vi "Autonomous Independent_old.vi"() -> ()   [LabVIEW 2011]
doc: "This VI is called when autonomous begins, and will automatically be terminated when autonomous ends. You can carry out timed or sensor driven robot movement independently without needing to return to the caller."
uses:
  <vilib>/Rock Robotics/WPI/Joystick/WPI_JoystickButtonState.ctl
  Robot Global Data.vi
  <vilib>/addons/control/pid/pid.llb/PID (DBL).vi
  <vilib>/Rock Robotics/WPI/RobotDrive/WPI_RobotDriveArcadeDrive_Standard(NoSaturation).vi
  <vilib>/addons/control/pid/NI_PID_pid.lvlib
panel:
  in  "ARM_FWD_LIMIT":dbl(slide)=0.4723926380368098 scale=1.0..-1.0
  in  "ARM_REV_LIMIT":dbl(slide)=-0.15950920245398775 scale=1.0..-1.0
  in  "ARM_HOME":dbl(slide)=0.47 scale=1.0..-1.0
  out "Kinect_Drive_Reduce":dbl=0.5
  out "KINECT_BTNS":T1
  out "LEFT_ARM_AXES":T2
  out "RIGHT_ARM_AXES":T2
  in  "Ball_Sucker_Speed":dbl=1.0
  in  "Feed_Speed_Cntrl":dbl=1.0
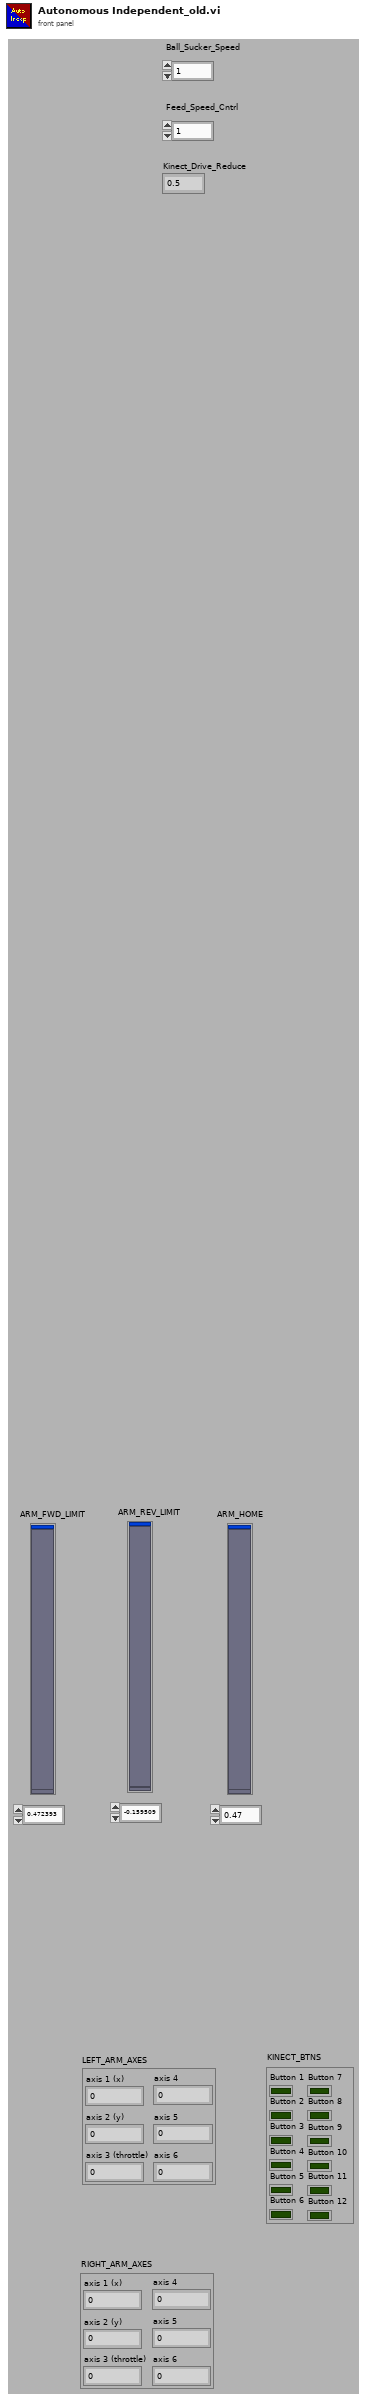
[diagram p1: front panel]
types:
  T1 = typedef "WPI_JoystickButtonState.ctl" = cluster{"Button 1":bool, "Button 2":bool, "Button 3":bool, "Button 4":bool, "Button 5":bool, "Button 6":bool, "Button 7":bool, "Button 8":bool, "Button 9":bool, "Button 10":bool, "Button 11":bool, "Button 12":bool}
  T2 = cluster{"axis 1 (x)":dbl, "axis 2 (y)":dbl, "axis 3 (throttle)":dbl, "axis 4":dbl, "axis 5":dbl, "axis 6":dbl}
  T3 = cluster{"proportional gain (Kc)":dbl, "integral time (Ti, min)":dbl, "derivative time (Td, min)":dbl}
  T4 = typedef "WPI_RobotDriveDevRef.ctl" = cluster{"DevStatus":errorcluster, "Motors[]":T5[], "Square Inputs":bool, "Max Output":dbl, "Isochronous":bool}
  T5 = typedef "WPI_MotorControlDeviceRef.ctl" = cluster{"DeviceStatus":errorcluster, "Type":enum16{"PWM", "CAN"}, "PWM":cluster{"Digital Module":T6, "PWM Channel":T7, "DeadBand":T8}, "CAN":cluster{"Device Number":u8, "Control Mode":T9, "Semaphore":T10, "Max Vout":dbl}, "Invert":bool, "TransformRef":T11, "InvTransformRef":T11}
  T6 = typedef "FPGA_TypedefDigitalModule.ctl" = enum16{"Digital Module 1", "Digital Module 2"}
  T7 = typedef "FPGA_DIOPWMChannel.ctl" = enum8{"PWM 1", "PWM 2", "PWM 3", "PWM 4", "PWM 5", "PWM 6", "PWM 7", "PWM 8", "PWM 9", "PWM 10", "Invalid"}
  T8 = typedef "WPI_PWMDeadband.ctl" = cluster{"Name":string, "maxPositivePwm":i32, "minPositivePwm":i32, "centerPwm":i32, "maxNegativePwm":i32, "minNegativePwm":i32, "angularRange":u16}
  T9 = typedef "WPI_CANJaguar_ControlMode.ctl" = enum8{"Percent VBus", "Current", "Speed", "Position", "Voltage"}
  T10 = typedef "Semaphore RefNum" = refnum<k1>
  T11 = typedef "WPI_PWMTransform_ConPane.ctl" = refnum<vi>
  T12 = typedef "WPI_JoystickDevRef.ctl" = cluster{"Device":T13}
  T13 = typedef "WPI_JoystickDeviceEnum.ctl" = enum16{"USB 1", "USB 2", "USB 3", "USB 4", "Kinect 1", "Kinect 2"}
  T14 = typedef "WPI_AnalogChannelDevRef.ctl" = cluster{"DevStatus":errorcluster, "Analog Module":T15, "Analog Channel":T16}
  T15 = typedef "FPGA_TypedefAnalogModule.ctl" = enum16{"Analog Module 1", "Analog Module 2"}
  T16 = typedef "FPGA_AIChannel.ctl" = enum8{"AI 1", "AI 2", "AI 3", "AI 4", "AI 5", "AI 6", "AI 7", "AI 8", "Invalid"}
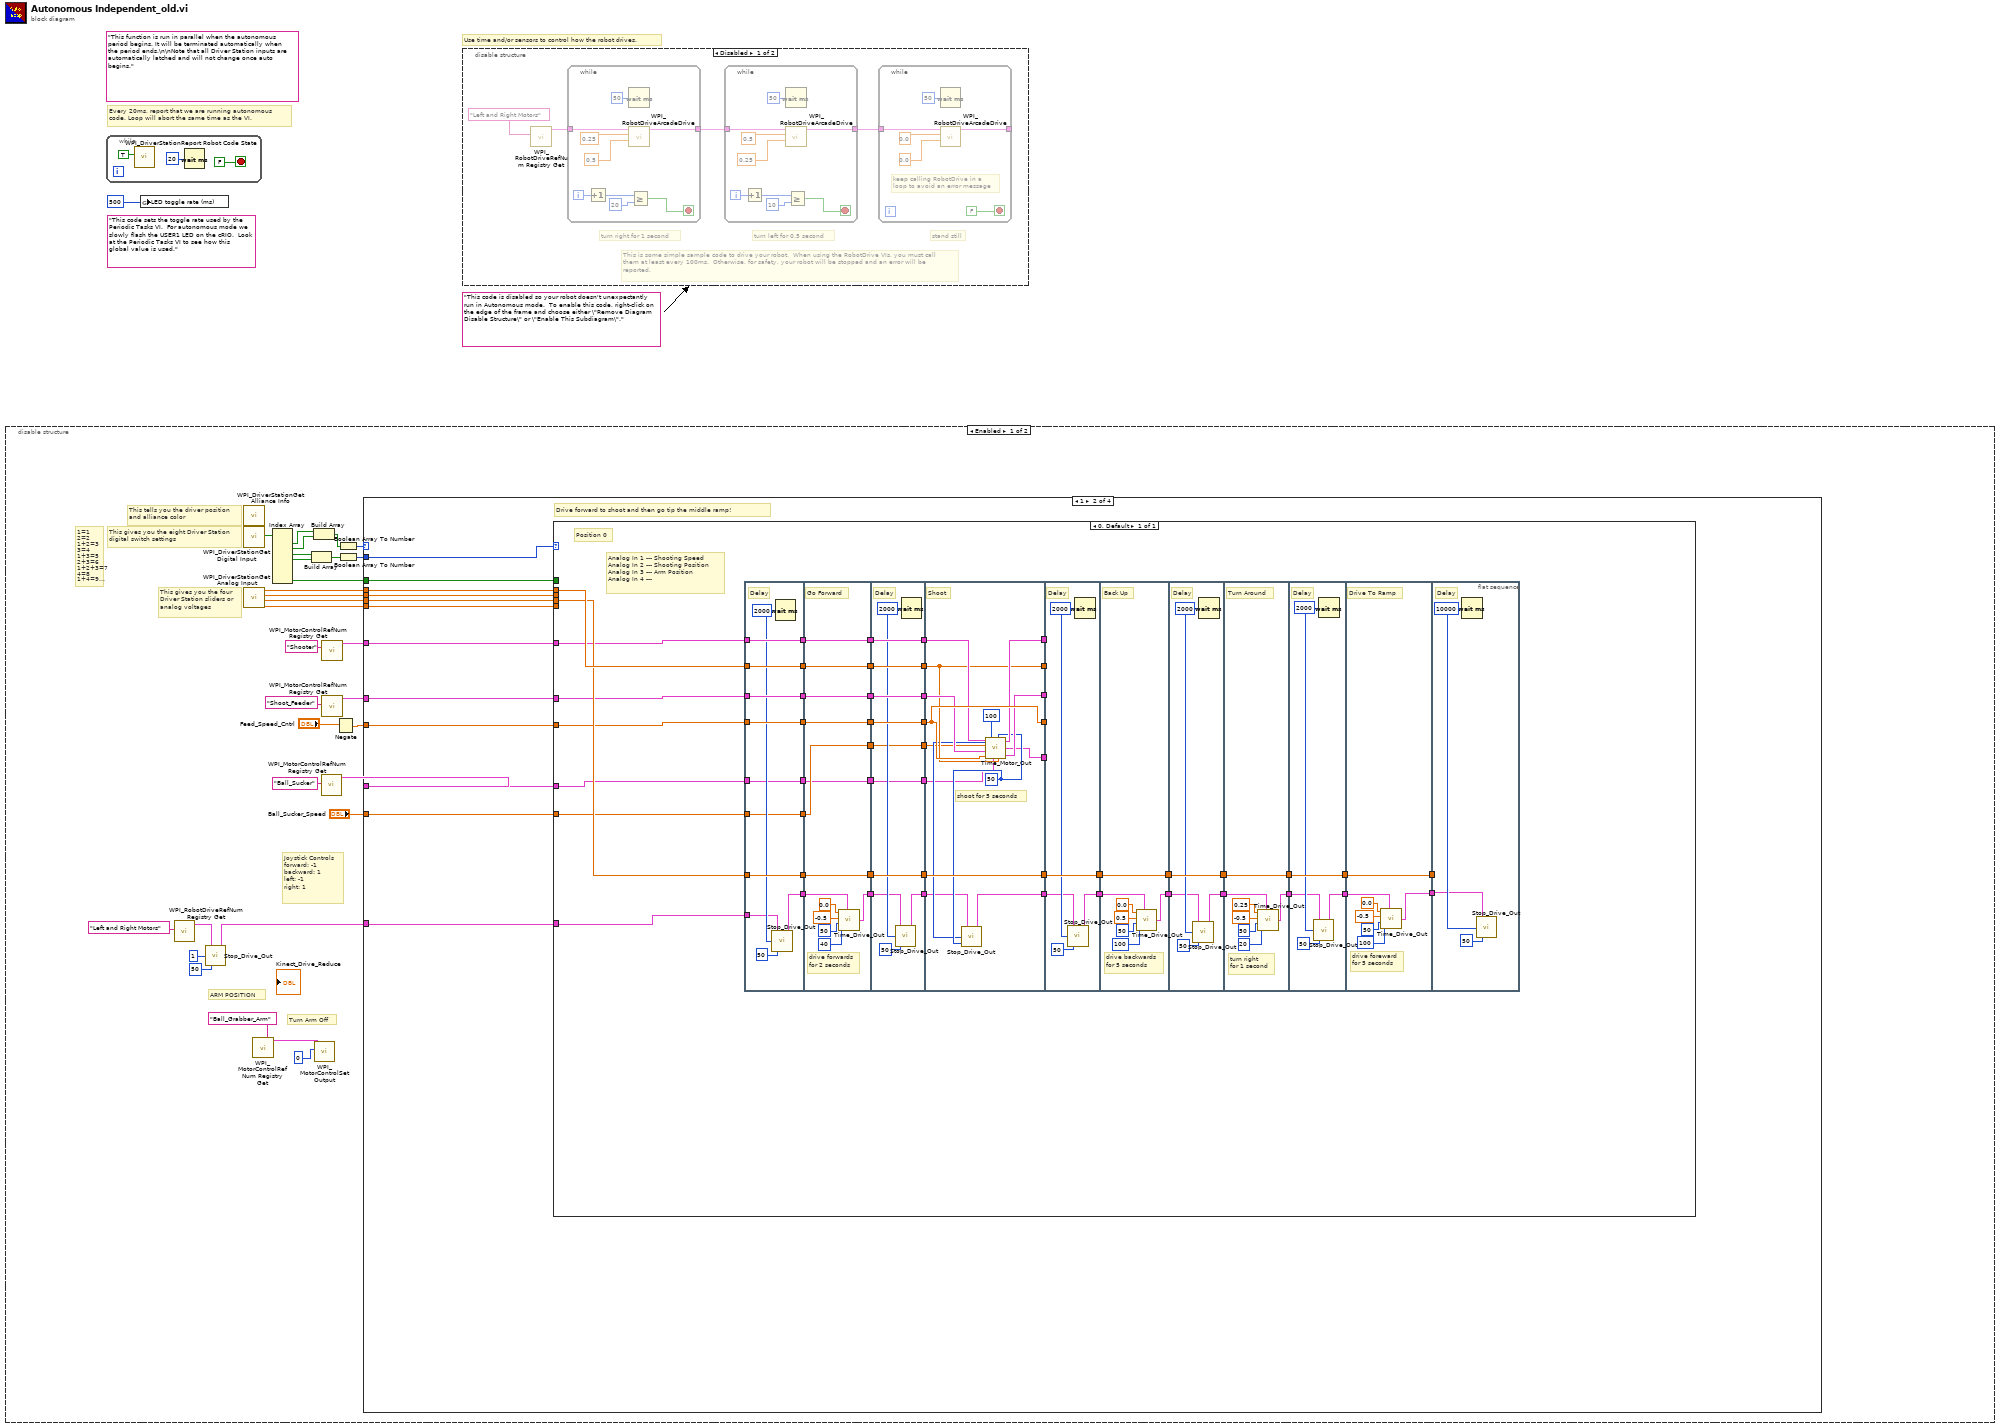
[diagram p0: block diagram]
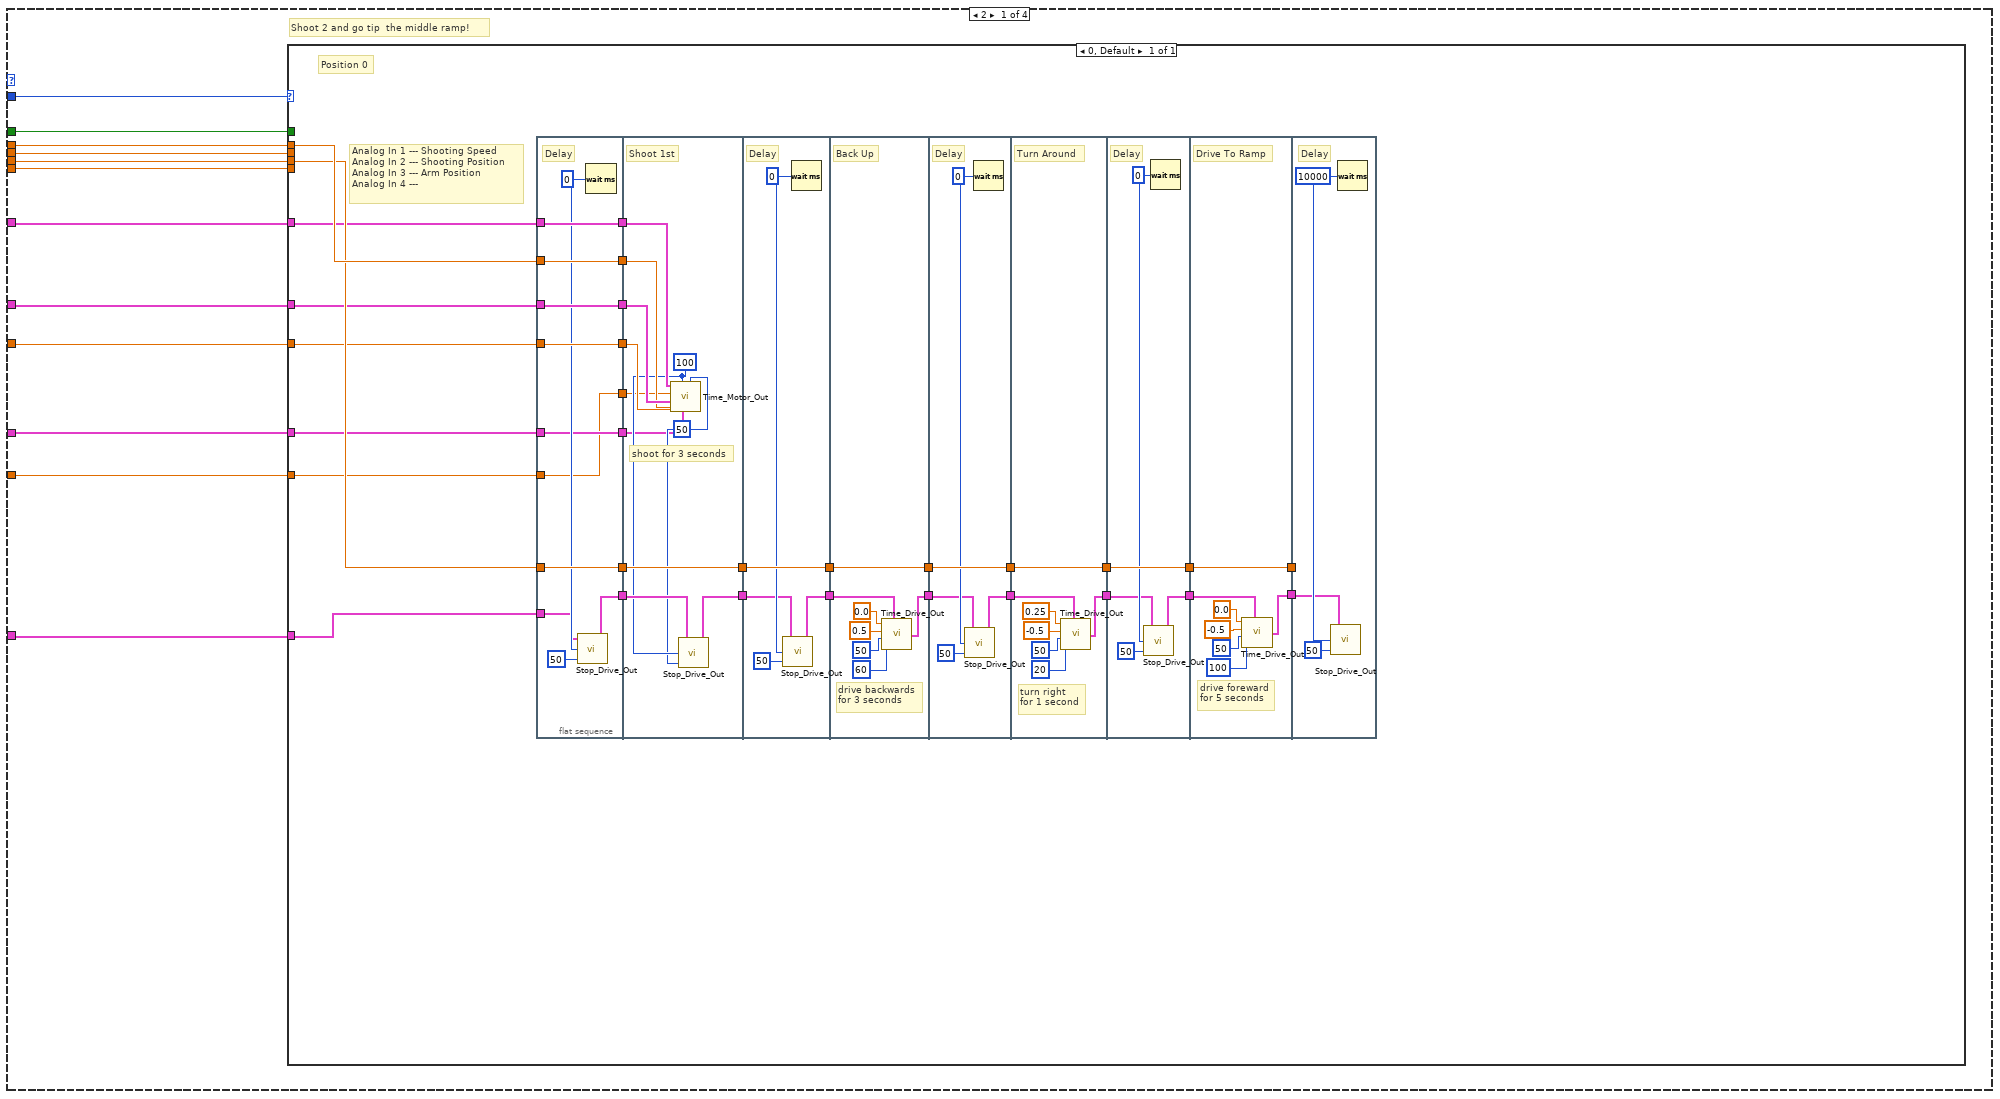
[diagram p2: hidden frame]
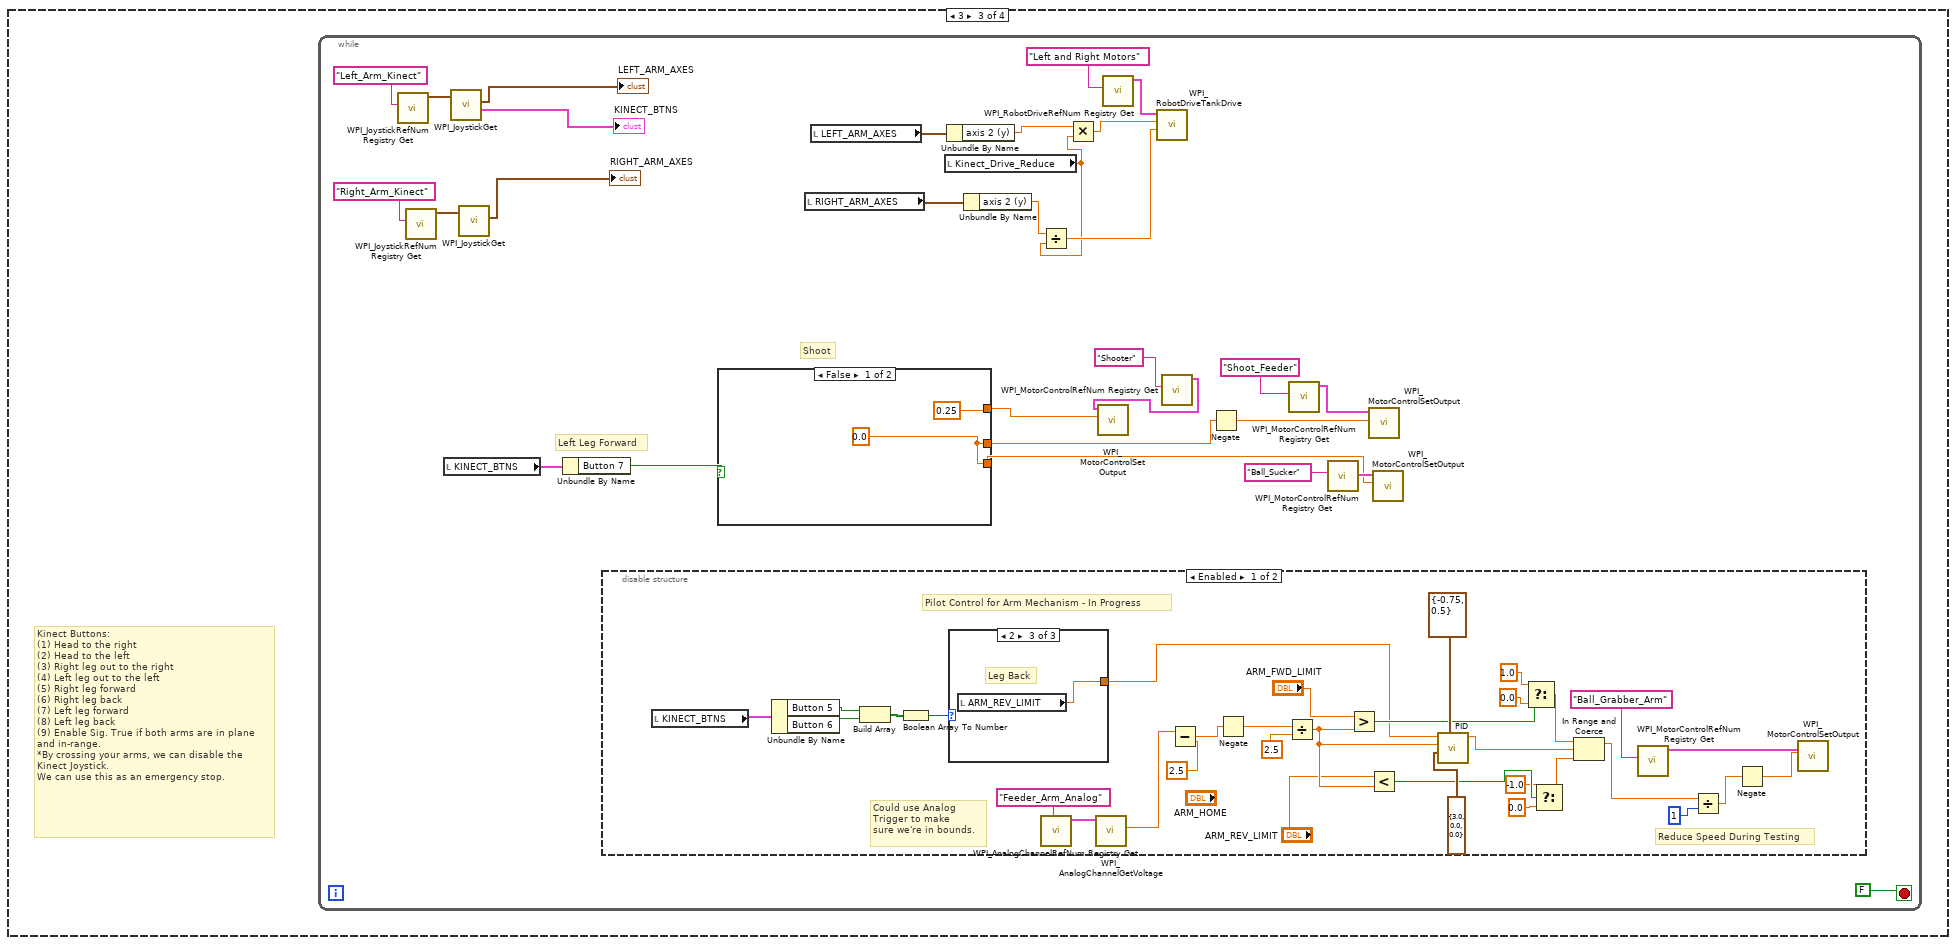
[diagram p3: hidden frame]
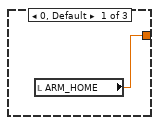
[diagram p4: hidden frame]
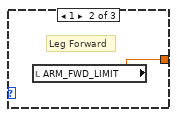
[diagram p5: hidden frame]
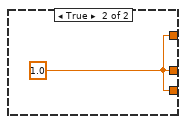
[diagram p7: hidden frame]
diagram:
  (unwired) "This code sets the toggle rate used by the Periodic Tasks VI.  For autonomous mode we slowly flash the USER1 LED on the cRIO.  Look at the Periodic Tasks VI to see how this global value is used."
  (unwired) "This code is disabled so your robot doesn't unexpectantly run in Autonomous mode.  To enable this code, right-click on the edge of the frame and choose either \"Remove Diagram Disable Structure\" or \"Enable This Subdiagram\"."
  (unwired) "This function is run in parallel when the autonomous period begins. It will be terminated automatically when the period ends.\n\nNote that all Driver Station inputs are automatically latched and will not change once auto begins."
  # "Every 20ms, report that we are running autonomous\ncode. Loop will abort the same time as the VI."
  # "Use time and/or sensors to control how the robot drives."
  n1 = disable-structure shown="Enabled" {
    frame Enabled {
      # "Turn Arm Off"
      # "ARM POSITION"
      # "Joystick Controls\nforward: -1\nbackward: 1\nleft: -1\nright: 1"
      # "1=1\n2=2\n1+2=3\n3=4\n1+3=5\n2+3=6\n1+2+3=7\n4=8\n1+4=9\n2+4=10\n1+2+4=11\n3+4=12\n1+3+4=13\n2+3+4=14\n1+2+3+4=15"
      # "This tells you the driver position\nand alliance color"
      # "This gives you the eight Driver Station\ndigital switch settings"
      # "This gives you the four\nDriver Station sliders or\nanalog voltages"
      n2 = call <vilib>:"WPI_RobotDriveRefNum Registry Get.vi"("refnum name"="Left and Right Motors") -> ("RobotDriveDevRef"=w13:T4)  [unwired: 1 in, 9 out]
      n3 = call "Stop_Drive_Out.vi"("Step_Duration_ms"=50, "Num_Steps"=u32 1 ("milliseconds to wait"), "Drive_In"=w13) -> ("Drive_Out"=w12:T4)
      n4 = call <vilib>:"WPI_DriverStationGet Alliance Info.vi"() -> ()  [unwired: 12 out]
      n5 = call <vilib>:"WPI_DriverStationGet Digital Input.vi"() -> ("Driver Station Digital Input (1-8)"=w32:bool[])  [unwired: 11 out]
      n6 = call <vilib>:"WPI_DriverStationGet Analog Input.vi"() -> ("Analog 4 (V)"=w29:dbl, "Analog 3 (V)"=w30:dbl, "Analog 2 (V)"=w16:dbl, "Analog 1 (V)"=w17:dbl)  [unwired: 8 out]
      n7 = call <vilib>:"WPI_MotorControlRefNum Registry Get.vi"("refnum name"="Ball_Grabber_Arm") -> ("MotorControlDevRef"=w4:T5)  [unwired: 1 in, 9 out]
      n8 = Index Array(array=w32) -> (element #1=w20:bool, element #2=w19:bool, element #3=w22:bool, element #4=w21:bool, element #8=w28:bool)  [unwired: 8 in, 3 out]
      n9 = Build Array(w22, w21) -> (w31:bool[])
      n10 = Build Array(w20, w19) -> (w18:bool[])
      n11 = call <vilib>:"WPI_MotorControlSetOutput.vi"("Output"=0, "MotorControlDevRef"=w4) -> ()  [unwired: 3 in, 7 out]
      n12 = call <vilib>:"WPI_MotorControlRefNum Registry Get.vi"("refnum name"="Ball_Sucker") -> ("MotorControlDevRef"=w6:T5)  [unwired: 9 in, 1 out]
      n13 = call <vilib>:"WPI_MotorControlRefNum Registry Get.vi"("refnum name"="Shooter") -> ("MotorControlDevRef"=w26:T5)  [unwired: 9 in, 1 out]
      n14 = call <vilib>:"WPI_MotorControlRefNum Registry Get.vi"("refnum name"="Shoot_Feeder") -> ("MotorControlDevRef"=w24:T5)  [unwired: 9 in, 1 out]
      n15 = Negate(x="Feed_Speed_Cntrl") -> (-x=w8:dbl)
      n16 = Boolean Array To Number(Boolean array=w18) -> (number=w11:u32)
      n17 = Boolean Array To Number(Boolean array=w31) -> (number=w10:u32)
      n18 = case shown="1" w11 {
        tunnel: w17 -> [w43 w146 _ _]
        tunnel: w16 -> [w42 w145 _ _]
        tunnel: w30 -> [w41 w144 _ _]
        tunnel: w29 -> [w40 w143 _ _]
        tunnel: w28 -> [w44 w147 _ _]
        tunnel: w8 -> [w39 w142 _ _]
        tunnel: w26 -> [w38 w141 _ _]
        tunnel: w24 -> [w37 w140 _ _]
        tunnel: w12 -> [w36 w139 _ _]
        tunnel: w10 -> [w35 w138 _ _]
        tunnel: w6 -> [w34 w137 _ _]
        tunnel: "Ball_Sucker_Speed" -> [w33 w136 _ _]
        frame 2 {
          # "Shoot 2 and go tip  the middle ramp!"
          n19 = case shown="0, Default" w35 {
            tunnel: w44 -> [_]
            tunnel: w43 -> [w74]
            tunnel: w42 -> [_]
            tunnel: w41 -> [w73]
            tunnel: w40 -> [_]
            tunnel: w39 -> [w72]
            tunnel: w38 -> [w71]
            tunnel: w37 -> [w70]
            tunnel: w36 -> [w69]
            tunnel: w34 -> [w45]
            tunnel: w33 -> [w68]
            frame 0, Default {
              # "Analog In 1 --- Shooting Speed\nAnalog In 2 --- Shooting Position\nAnalog In 3 --- Arm Position\nAnalog In 4 ---"
              # "Position 0"
              n20 = flat-sequence {
                tunnel: [w85] -> w67
                tunnel: [w84] -> w66
                tunnel: [w80] -> w65
                tunnel: [w83] -> w64
                tunnel: [w82] -> w63
                tunnel: [w81] -> w62
                tunnel: w71 -> [w85]
                tunnel: w70 -> [w84]
                tunnel: w74 -> [w83]
                tunnel: w72 -> [w82]
                tunnel: w73 -> [w81]
                tunnel: w69 -> [w77]
                tunnel: w45 -> [w76]
                tunnel: [w76] -> w61
                tunnel: [w75] -> w60
                tunnel: w68 -> [w75]
                tunnel: w67 -> [w96]
                tunnel: w66 -> [w95]
                tunnel: w65 -> [w91]
                tunnel: w64 -> [w93]
                tunnel: w63 -> [w94]
                tunnel: [w92] -> w59
                tunnel: w62 -> [w92]
                tunnel: [w88] -> w58
                tunnel: w61 -> [w87]
                tunnel: w60 -> [w86]
                tunnel: [w98] -> w57
                tunnel: [w101] -> w56
                tunnel: w59 -> [w101]
                tunnel: w58 -> [w97]
                tunnel: w57 -> [w104]
                tunnel: [w103] -> w55
                tunnel: w56 -> [w102]
                tunnel: [w102] -> w54
                tunnel: w55 -> [w110]
                tunnel: [w113] -> w53
                tunnel: w54 -> [w113]
                tunnel: [w109] -> w52
                tunnel: [w115] -> w51
                tunnel: [w114] -> w50
                tunnel: w53 -> [w114]
                tunnel: w52 -> [w116]
                tunnel: w51 -> [w122]
                tunnel: [w125] -> w49
                tunnel: w50 -> [w125]
                tunnel: [w121] -> w48
                tunnel: [w127] -> w47
                tunnel: [w126] -> w46
                tunnel: w49 -> [w126]
                tunnel: w48 -> [w128]
                tunnel: w47 -> [w133]
                tunnel: w46 -> [_]
                frame #0 {
                  w79 = u32 0 ("milliseconds to wait")
                  # "Delay"
                  n21 = call "Stop_Drive_Out.vi"("Step_Duration_ms"=u32 50 ("milliseconds to wait"), "Num_Steps"=w79, "Drive_In"=w77) -> ("Drive_Out"=w80:T4)
                  n22 = Wait (ms)(milliseconds to wait=w79) -> ()  [unwired: 1 out]
                }
                frame #1 {
                  w89 = 50
                  w90 = 100
                  # "shoot for 3 seconds"
                  # "Shoot 1st"
                  n23 = call "Time_Motor_Out.vi"("Motor_1_Speed"=w93, "Step_Duration_ms"=w89, "Motor_3"=w87, "Motor_2_Speed"=w94, "Motor_2"=w95, "Num_Steps"=w90, "Motor_3_Speed"=w86, "Motor_1"=w96) -> ()  [unwired: 3 out]
                  n24 = call "Stop_Drive_Out.vi"("Step_Duration_ms"=w89, "Num_Steps"=w90, "Drive_In"=w91) -> ("Drive_Out"=w88:T4)
                }
                frame #2 {
                  w99 = u32 0 ("milliseconds to wait")
                  # "Delay"
                  n25 = call "Stop_Drive_Out.vi"("Step_Duration_ms"=u32 50 ("milliseconds to wait"), "Num_Steps"=w99, "Drive_In"=w97) -> ("Drive_Out"=w98:T4)
                  n26 = Wait (ms)(milliseconds to wait=w99) -> ()  [unwired: 1 out]
                }
                frame #3 {
                  # "drive backwards\nfor 3 seconds"
                  # "Back Up"
                  n27 = call "Time_Drive_Out.vi"("X_Axis"=0.0 ("X axis value"), "Y_Axis"=0.5 ("X axis value"), "Step_Duration_ms"=u32 50 ("milliseconds to wait"), "Num_Steps"=60, "Drive_In"=w104) -> ("Drive_Out"=w103:T4)
                }
                frame #4 {
                  w111 = u32 0 ("milliseconds to wait")
                  # "Delay"
                  n28 = call "Stop_Drive_Out.vi"("Step_Duration_ms"=u32 50 ("milliseconds to wait"), "Num_Steps"=w111, "Drive_In"=w110) -> ("Drive_Out"=w109:T4)
                  n29 = Wait (ms)(milliseconds to wait=w111) -> ()  [unwired: 1 out]
                }
                frame #5 {
                  # "turn right\nfor 1 second"
                  # "Turn Around"
                  n30 = call "Time_Drive_Out.vi"("X_Axis"=0.25 ("X axis value"), "Y_Axis"=-0.5 ("X axis value"), "Step_Duration_ms"=u32 50 ("milliseconds to wait"), "Num_Steps"=20, "Drive_In"=w116) -> ("Drive_Out"=w115:T4)
                }
                frame #6 {
                  w123 = u32 0 ("milliseconds to wait")
                  # "Delay"
                  n31 = call "Stop_Drive_Out.vi"("Step_Duration_ms"=u32 50 ("milliseconds to wait"), "Num_Steps"=w123, "Drive_In"=w122) -> ("Drive_Out"=w121:T4)
                  n32 = Wait (ms)(milliseconds to wait=w123) -> ()  [unwired: 1 out]
                }
                frame #7 {
                  # "drive foreward\nfor 5 seconds"
                  # "Drive To Ramp"
                  n33 = call "Time_Drive_Out.vi"("X_Axis"=0.0 ("X axis value"), "Y_Axis"=-0.5 ("X axis value"), "Step_Duration_ms"=u32 50 ("milliseconds to wait"), "Num_Steps"=100, "Drive_In"=w128) -> ("Drive_Out"=w127:T4)
                }
                frame #8 {
                  w134 = u32 10000 ("milliseconds to wait")
                  # "Delay"
                  n34 = call "Stop_Drive_Out.vi"("Step_Duration_ms"=u32 50 ("milliseconds to wait"), "Num_Steps"=w134, "Drive_In"=w133) -> ()  [unwired: 1 out]
                  n35 = Wait (ms)(milliseconds to wait=w134) -> ()  [unwired: 1 out]
                }
              }
            }
          }
        }
        frame 1 {
          # "Drive forward to shoot and then go tip the middle ramp!"
          n36 = case shown="0, Default" w138 {
            tunnel: w147 -> [_]
            tunnel: w146 -> [w198]
            tunnel: w145 -> [_]
            tunnel: w144 -> [w197]
            tunnel: w143 -> [_]
            tunnel: w142 -> [w196]
            tunnel: w141 -> [w195]
            tunnel: w140 -> [w194]
            tunnel: w139 -> [w193]
            tunnel: w137 -> [w192]
            tunnel: w136 -> [w191]
            frame 0, Default {
              # "Analog In 1 --- Shooting Speed\nAnalog In 2 --- Shooting Position\nAnalog In 3 --- Arm Position\nAnalog In 4 ---"
              # "Position 0"
              n37 = flat-sequence {
                tunnel: [w202] -> w190
                tunnel: [w209] -> w189
                tunnel: [w208] -> w188
                tunnel: [w207] -> w187
                tunnel: [w206] -> w186
                tunnel: [w205] -> w185
                tunnel: w195 -> [w207]
                tunnel: w194 -> [w208]
                tunnel: w198 -> [w206]
                tunnel: w196 -> [w209]
                tunnel: w197 -> [w205]
                tunnel: w193 -> [w201]
                tunnel: [w200] -> w184
                tunnel: w191 -> [w200]
                tunnel: [w199] -> w183
                tunnel: w192 -> [w199]
                tunnel: w190 -> [w218]
                tunnel: [w217] -> w182
                tunnel: [w216] -> w181
                tunnel: w189 -> [w216]
                tunnel: [w215] -> w180
                tunnel: w188 -> [w215]
                tunnel: [w214] -> w179
                tunnel: w187 -> [w214]
                tunnel: [w213] -> w178
                tunnel: w186 -> [w213]
                tunnel: w185 -> [w212]
                tunnel: [w212] -> w177
                tunnel: w184 -> [w211]
                tunnel: [w211] -> w176
                tunnel: w183 -> [w210]
                tunnel: [w210] -> w175
                tunnel: w182 -> [w226]
                tunnel: [w225] -> w174
                tunnel: [w233] -> w173
                tunnel: [w232] -> w172
                tunnel: w181 -> [w232]
                tunnel: [w231] -> w171
                tunnel: w180 -> [w231]
                tunnel: [w230] -> w170
                tunnel: w179 -> [w230]
                tunnel: [w229] -> w169
                tunnel: w178 -> [w229]
                tunnel: w177 -> [w233]
                tunnel: [w224] -> w168
                tunnel: w176 -> [w224]
                tunnel: [w223] -> w167
                tunnel: w175 -> [w223]
                tunnel: w174 -> [w238]
                tunnel: [w237] -> w166
                tunnel: w173 -> [w247]
                tunnel: [w247] -> w165
                tunnel: w172 -> [w246]
                tunnel: [w246] -> w164
                tunnel: w171 -> [w245]
                tunnel: [w244] -> w163
                tunnel: [w243] -> w162
                tunnel: w170 -> [w242]
                tunnel: w169 -> [w241]
                tunnel: [w241] -> w161
                tunnel: [w236] -> w160
                tunnel: w168 -> [w235]
                tunnel: w167 -> [w234]
                tunnel: w166 -> [w249]
                tunnel: [w248] -> w159
                tunnel: w165 -> [w252]
                tunnel: [w252] -> w158
                tunnel: w164 -> [_]
                tunnel: w163 -> [_]
                tunnel: w162 -> [_]
                tunnel: w161 -> [_]
                tunnel: w160 -> [_]
                tunnel: w159 -> [w254]
                tunnel: [w253] -> w157
                tunnel: w158 -> [w259]
                tunnel: [w259] -> w156
                tunnel: w157 -> [w261]
                tunnel: w156 -> [w264]
                tunnel: [w264] -> w155
                tunnel: [w260] -> w154
                tunnel: [w266] -> w153
                tunnel: [w265] -> w152
                tunnel: w155 -> [w265]
                tunnel: w154 -> [w267]
                tunnel: w153 -> [w273]
                tunnel: [w272] -> w151
                tunnel: [w276] -> w150
                tunnel: w152 -> [w276]
                tunnel: w151 -> [w279]
                tunnel: [w278] -> w149
                tunnel: [w277] -> w148
                tunnel: w150 -> [w277]
                tunnel: w149 -> [w284]
                tunnel: w148 -> [_]
                frame #0 {
                  w203 = u32 2000 ("milliseconds to wait")
                  # "Delay"
                  n38 = call "Stop_Drive_Out.vi"("Step_Duration_ms"=50, "Num_Steps"=w203, "Drive_In"=w201) -> ("Drive_Out"=w202:T4)
                  n39 = Wait (ms)(milliseconds to wait=w203) -> ()  [unwired: 1 out]
                }
                frame #1 {
                  # "drive forwards\nfor 2 seconds"
                  # "Go Forward"
                  n40 = call "Time_Drive_Out.vi"("X_Axis"=0.0 ("X axis value"), "Y_Axis"=-0.5 ("X axis value"), "Step_Duration_ms"=u32 50 ("milliseconds to wait"), "Num_Steps"=40, "Drive_In"=w218) -> ("Drive_Out"=w217:T4)
                }
                frame #2 {
                  w227 = u32 2000 ("milliseconds to wait")
                  # "Delay"
                  n41 = call "Stop_Drive_Out.vi"("Step_Duration_ms"=50, "Num_Steps"=w227, "Drive_In"=w226) -> ("Drive_Out"=w225:T4)
                  n42 = Wait (ms)(milliseconds to wait=w227) -> ()  [unwired: 1 out]
                }
                frame #3 {
                  w240 = 50
                  w239 = 100
                  # "Shoot"
                  # "shoot for 5 seconds"
                  n43 = call "Stop_Drive_Out.vi"("Step_Duration_ms"=w240, "Num_Steps"=w239, "Drive_In"=w238) -> ("Drive_Out"=w237:T4)
                  n44 = call "Time_Motor_Out.vi"("Motor_1_Speed"=w241, "Step_Duration_ms"=w240, "Motor_3"=w234, "Motor_2_Speed"=w246, "Motor_2"=w245, "Num_Steps"=w239, "Motor_3_Speed"=w235, "Motor_1"=w242) -> ("Motor_2_Out"=w244:T5, "Motor_3_Out"=w236:T5, "Motor_1_Out"=w243:T5)
                }
                frame #4 {
                  w250 = u32 2000 ("milliseconds to wait")
                  # "Delay"
                  n45 = call "Stop_Drive_Out.vi"("Step_Duration_ms"=50, "Num_Steps"=w250, "Drive_In"=w249) -> ("Drive_Out"=w248:T4)
                  n46 = Wait (ms)(milliseconds to wait=w250) -> ()  [unwired: 1 out]
                }
                frame #5 {
                  # "Back Up"
                  # "drive backwards\nfor 5 seconds"
                  n47 = call "Time_Drive_Out.vi"("X_Axis"=0.0 ("X axis value"), "Y_Axis"=0.5 ("X axis value"), "Step_Duration_ms"=u32 50 ("milliseconds to wait"), "Num_Steps"=100, "Drive_In"=w254) -> ("Drive_Out"=w253:T4)
                }
                frame #6 {
                  w262 = u32 2000 ("milliseconds to wait")
                  # "Delay"
                  n48 = call "Stop_Drive_Out.vi"("Step_Duration_ms"=50, "Num_Steps"=w262, "Drive_In"=w261) -> ("Drive_Out"=w260:T4)
                  n49 = Wait (ms)(milliseconds to wait=w262) -> ()  [unwired: 1 out]
                }
                frame #7 {
                  # "turn right\nfor 1 second"
                  # "Turn Around"
                  n50 = call "Time_Drive_Out.vi"("X_Axis"=0.25 ("X axis value"), "Y_Axis"=-0.5 ("X axis value"), "Step_Duration_ms"=u32 50 ("milliseconds to wait"), "Num_Steps"=20, "Drive_In"=w267) -> ("Drive_Out"=w266:T4)
                }
                frame #8 {
                  w274 = u32 2000 ("milliseconds to wait")
                  # "Delay"
                  n51 = call "Stop_Drive_Out.vi"("Step_Duration_ms"=50, "Num_Steps"=w274, "Drive_In"=w273) -> ("Drive_Out"=w272:T4)
                  n52 = Wait (ms)(milliseconds to wait=w274) -> ()  [unwired: 1 out]
                }
                frame #9 {
                  # "drive foreward\nfor 5 seconds"
                  # "Drive To Ramp"
                  n53 = call "Time_Drive_Out.vi"("X_Axis"=0.0 ("X axis value"), "Y_Axis"=-0.5 ("X axis value"), "Step_Duration_ms"=u32 50 ("milliseconds to wait"), "Num_Steps"=100, "Drive_In"=w279) -> ("Drive_Out"=w278:T4)
                }
                frame #10 {
                  w285 = u32 10000 ("milliseconds to wait")
                  # "Delay"
                  n54 = Wait (ms)(milliseconds to wait=w285) -> ()  [unwired: 1 out]
                  n55 = call "Stop_Drive_Out.vi"("Step_Duration_ms"=50, "Num_Steps"=w285, "Drive_In"=w284) -> ()  [unwired: 1 out]
                }
              }
            }
          }
        }
        frame 3 {
          # "Kinect Buttons:\n(1) Head to the right\n(2) Head to the left\n(3) Right leg out to the right\n(4) Left leg out to the left\n(5) Right leg forward\n(6) Right leg back\n(7) Left leg forward\n(8) Left leg back\n(9) Enable Sig. True if both arms are in plane and in-range.\n*By crossing your arms, we can disable the Kinect Joystick. \nWe can use this as an emergency stop."
          n56 = while {
            stop <- FALSE stop-if-true
            # "Left Leg Forward"
            # "Shoot"
            n57 = call <vilib>:"WPI_JoystickRefNum Registry Get.vi"("refnum name"="Left_Arm_Kinect") -> ("JoystickDevRef"=w312:T12)  [unwired: 1 in, 9 out]
            n58 = call <vilib>:"WPI_JoystickRefNum Registry Get.vi"("refnum name"="Right_Arm_Kinect") -> ("JoystickDevRef"=w310:T12)  [unwired: 1 in, 9 out]
            n59 = local read "KINECT_BTNS"() -> (w299:T1)
            n60 = call <vilib>:"WPI_JoystickGet.vi"("JoystickDevRef"=w312) -> ("Buttons"=→"KINECT_BTNS":T1, "Axes"=→"LEFT_ARM_AXES":T2)  [unwired: 1 in, 4 out]
            n61 = call <vilib>:"WPI_JoystickGet.vi"("JoystickDevRef"=w310) -> ("Axes"=→"RIGHT_ARM_AXES":T2)  [unwired: 1 in, 5 out]
            n62 = Unbundle By Name(w299) -> ("Button 7"=w298:bool)
            n63 = disable-structure shown="Enabled" {
              frame Enabled {
                # "Could use Analog\nTrigger to make \nsure we're in bounds."
                # "Reduce Speed During Testing"
                # "Pilot Control for Arm Mechanism - In Progress"
                n64 = local read "KINECT_BTNS"() -> (w320:T1)
                n65 = Unbundle By Name(w320) -> ("Button 5"=w317:bool, "Button 6"=w316:bool)
                n66 = Build Array(w317, w316) -> (w318:bool[])
                n67 = Boolean Array To Number(Boolean array=w318) -> (number=w319:u32)
                n68 = case shown="2" w319 {
                  tunnel: [w349 w350 w351] -> w326
                  frame 0, Default {
                    n69 = local read "ARM_HOME"() -> (w349:dbl)
                  }
                  frame 1 {
                    # "Leg Forward"
                    n70 = local read "ARM_FWD_LIMIT"() -> (w350:dbl)
                  }
                  frame 2 {
                    # "Leg Back"
                    n71 = local read "ARM_REV_LIMIT"() -> (w351:dbl)
                  }
                }
                n72 = call <vilib>:"WPI_AnalogChannelRefNum Registry Get.vi"("refnum name"="Feeder_Arm_Analog") -> ("AIDeviceRef"=w347:T14)  [unwired: 1 in, 9 out]
                n73 = call <vilib>:"WPI_AnalogChannelGetVoltage.vi"("AIDeviceRef"=w347) -> ("Voltage"=w344:dbl)  [unwired: 1 in, 9 out]
                n74 = Subtract(x=w344, y=2.5) -> (x-y=w321:dbl)
                n75 = Negate(x=w321) -> (-x=w322:dbl)
                n76 = Divide(x=w322, y=2.5) -> (x/y=w332:dbl)
                n77 = Greater?(x="ARM_FWD_LIMIT", y=w332) -> (0:w339:bool)
                n78 = Less?(x="ARM_REV_LIMIT", y=w332) -> (x < y?=w341:bool)
                n79 = call-poly <vilib>:"PID.vi"("output range"=cluster{"output low":dbl, "output high":dbl} {"output low"=-0.75, "output high"=0.5}, "PID gains"=T3 {"proportional gain (Kc)"=3.0, "integral time (Ti, min)"=0.0, "derivative time (Td, min)"=0.0}, "process variable"=w332, "setpoint"=w326) -> ("output"=w331:dbl)  [unwired: 2 in, 5 out]
                n80 = Select(t=1.0, s=w339, f=0.0) -> (s? t:f=w337:dbl)
                n81 = Select(t=-1.0, s=w341, f=0.0) -> (s? t:f=w338:dbl)
                n82 = In Range and Coerce(upper limit=w337, x=w331, lower limit=w338) -> (coerced(x)=w328:dbl)  [unwired: 1 out]
                n83 = call <vilib>:"WPI_MotorControlRefNum Registry Get.vi"("refnum name"="Ball_Grabber_Arm") -> ("MotorControlDevRef"=w348:T5)  [unwired: 1 in, 9 out]
                n84 = Divide(x=w328, y=1) -> (x/y=w324:dbl)
                n85 = Negate(x=w324) -> (-x=w323:dbl)
                n86 = call <vilib>:"WPI_MotorControlSetOutput.vi"("Output"=w323, "MotorControlDevRef"=w348) -> ()  [unwired: 3 in, 7 out]
              }
              frame Disabled {
              }
            }
            n87 = case shown="False" w298 {
              tunnel: [0.25 w354] -> w290
              tunnel: [w353 w354] -> w289
              tunnel: [w353 w354] -> w288
              frame False {
                w353 = 0.0
              }
              frame True {
                w354 = 1.0
              }
            }
            n88 = local read "RIGHT_ARM_AXES"() -> (w303:T2)
            n89 = local read "LEFT_ARM_AXES"() -> (w306:T2)
            n90 = local read "Kinect_Drive_Reduce"() -> (w300:dbl)
            n91 = Unbundle By Name(w306) -> ("axis 2 (y)"=w305:dbl)
            n92 = Unbundle By Name(w303) -> ("axis 2 (y)"=w302:dbl)
            n93 = Divide(x=w302, y=w300) -> (x/y=w301:dbl)
            n94 = Multiply(x=w305, y=w300) -> (x*y=w304:dbl)
            n95 = call <vilib>:"WPI_RobotDriveRefNum Registry Get.vi"("refnum name"="Left and Right Motors") -> ("RobotDriveDevRef"=w307:T4)  [unwired: 1 in, 9 out]
            n96 = call <vilib>:"WPI_RobotDriveTankDrive.vi"("Right axis value"=w301, "Left axis value"=w304, "RobotDriveDevRef"=w307) -> ()  [unwired: 7 in, 2 out]
            n97 = call <vilib>:"WPI_MotorControlRefNum Registry Get.vi"("refnum name"="Shooter") -> ("MotorControlDevRef"=w296:T5)  [unwired: 9 in, 1 out]
            n98 = call <vilib>:"WPI_MotorControlSetOutput.vi"("Output"=w290, "MotorControlDevRef"=w296) -> ()  [unwired: 8 in, 2 out]
            n99 = Negate(x=w289) -> (-x=w293:dbl)
            n100 = call <vilib>:"WPI_MotorControlRefNum Registry Get.vi"("refnum name"="Shoot_Feeder") -> ("MotorControlDevRef"=w294:T5)  [unwired: 9 in, 1 out]
            n101 = call <vilib>:"WPI_MotorControlRefNum Registry Get.vi"("refnum name"="Ball_Sucker") -> ("MotorControlDevRef"=w291:T5)  [unwired: 9 in, 1 out]
            n102 = call <vilib>:"WPI_MotorControlSetOutput.vi"("Output"=w293, "MotorControlDevRef"=w294) -> ()  [unwired: 8 in, 2 out]
            n103 = call <vilib>:"WPI_MotorControlSetOutput.vi"("Output"=w288, "MotorControlDevRef"=w291) -> ()  [unwired: 8 in, 2 out]
          }
        }
        frame 0, Default {
          # "Stop Motors"
        }
      }
    }
    frame Disabled {
    }
  }
  n104 = while {
    stop <- FALSE stop-if-true
    n105 = call <vilib>:"WPI_DriverStationReport Robot Code State.vi"("Autonomous"=TRUE) -> ()  [unwired: 10 in, 1 out]
    n106 = Wait (ms)(milliseconds to wait=u32 20) -> ()  [unwired: 1 out]
  }
  n107 = global write "Robot Global Data.vi" "LED toggle rate (ms)"(u32 500 ("LED ms toggle rate")) -> ()
  n108 = disable-structure shown="Disabled" {
    frame Disabled {
      # "This is some simple sample code to drive your robot.  When using the RobotDrive VIs, you must call them at least every 100ms.  Otherwise, for safety, your robot will be stopped and an error will be reported."
      # "stand still"
      # "turn left for 0.5 second"
      # "turn right for 1 second"
      n109 = call <vilib>:"WPI_RobotDriveRefNum Registry Get.vi"("refnum name"="Left and Right Motors") -> ("RobotDriveDevRef"=w360:T4)  [unwired: 1 in, 9 out]
      n110 = while {
        tunnel: w360 -> [w385]
        tunnel: [w378] -> w359
        i -> [w381]
        stop <- w379 stop-if-true
        n111 = Increment(x=w381) -> (x+1=w377:i32)
        n112 = Wait (ms)(milliseconds to wait=u32 50) -> ()  [unwired: 1 out]
        n113 = call-poly <vilib>:"WPI_RobotDriveArcadeDrive.vi"("Y axis value"=0.5 ("X axis value"), "X axis value"=0.25, "RobotDriveDevRef"=w385) -> ("RobotDriveDevRef"=w378:T4)  [unwired: 1 in, 7 out]
        n114 = Greater Or Equal?(x=w377, y=20) -> (x >= y?=w379:bool)
      }
      n115 = while {
        tunnel: w359 -> [w376]
        tunnel: [w369] -> w358
        i -> [w372]
        stop <- w370 stop-if-true
        n116 = Increment(x=w372) -> (x+1=w368:i32)
        n117 = Wait (ms)(milliseconds to wait=u32 50) -> ()  [unwired: 1 out]
        n118 = call-poly <vilib>:"WPI_RobotDriveArcadeDrive.vi"("Y axis value"=0.25 ("X axis value"), "X axis value"=0.5, "RobotDriveDevRef"=w376) -> ("RobotDriveDevRef"=w369:T4)  [unwired: 1 in, 7 out]
        n119 = Greater Or Equal?(x=w368, y=10) -> (x >= y?=w370:bool)
      }
      n120 = while {
        tunnel: w358 -> [w367]
        tunnel: [w363] -> _
        stop <- FALSE stop-if-true
        # "keep calling RobotDrive in a loop to avoid an error message"
        n121 = Wait (ms)(milliseconds to wait=u32 50) -> ()  [unwired: 1 out]
        n122 = call-poly <vilib>:"WPI_RobotDriveArcadeDrive.vi"("Y axis value"=0.0 ("X axis value"), "X axis value"=0.0, "RobotDriveDevRef"=w367) -> ("RobotDriveDevRef"=w363:T4)  [unwired: 1 in, 7 out]
      }
    }
    frame Enabled {
    }
  }
